vi "TEST Drop In.vi"(8 "error in (no error)":errorcluster, 10 "Queue Name":string="Main") -> (0 "error out":errorcluster)   [LabVIEW 2011]
doc: "This is the TEST VI that the user will leverage to test the drop in. \n\nAAL 9/09"
uses:
  Shared/QDMH Poly VIs/QDMH POLY Enqueue String.vi
panel:
  in  "Test 3":bool
  in  "Test 2":bool
  in  "Test 1":bool
  out "Message Display":string
  in  "Exit":bool
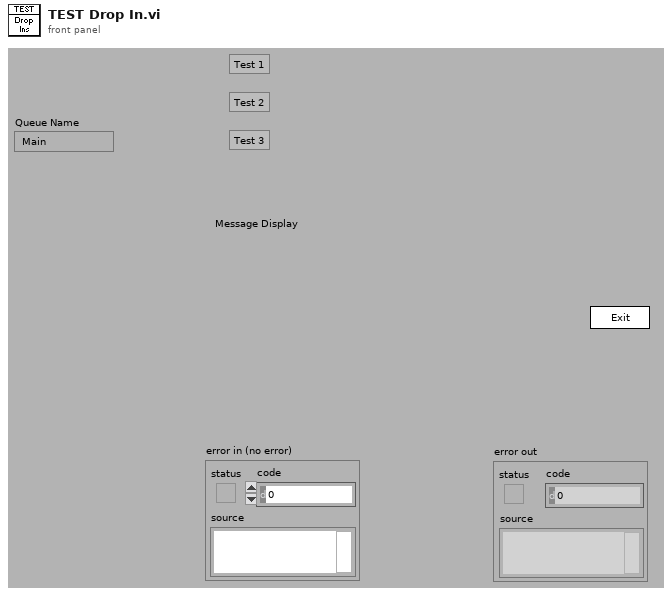
[diagram p1: front panel]
types:
  T1 = cluster{"Operator Name":string, "Current VI's Path":path, "Current VI's  Directory":path, "Queue Names":string[], "# VIs Launched":i32}
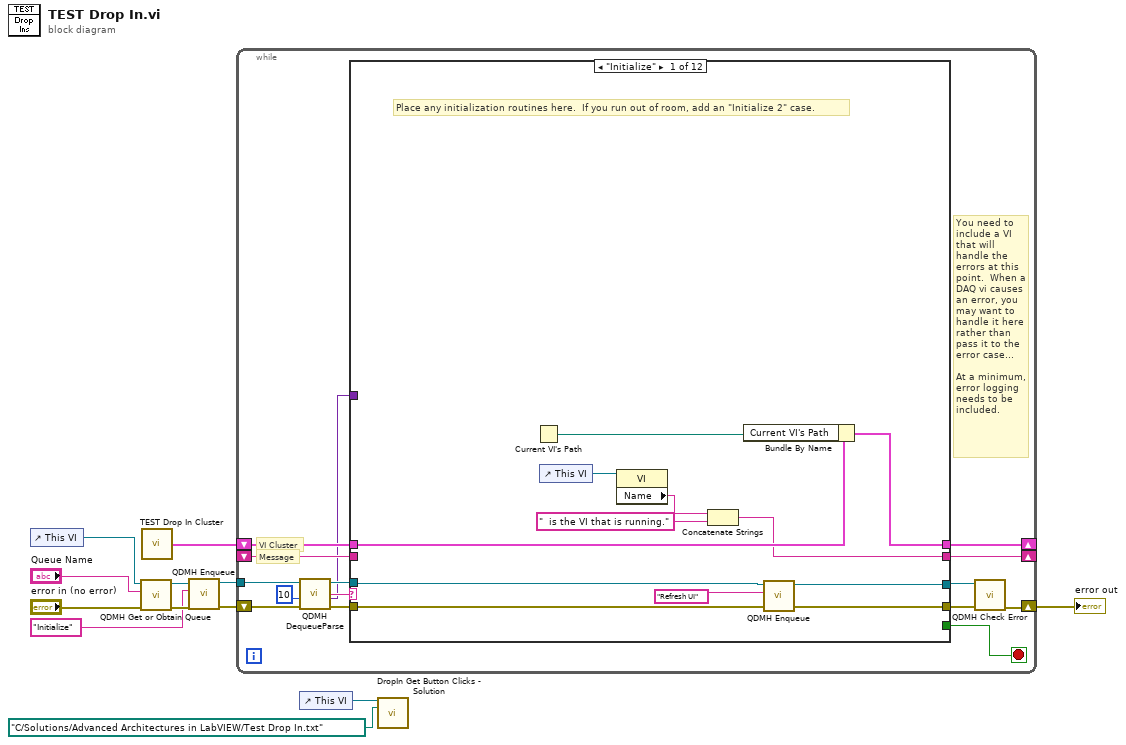
[diagram p0: block diagram]
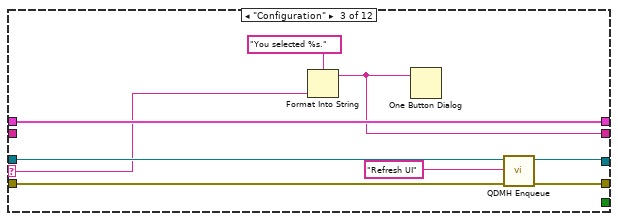
[diagram p3: hidden frame]
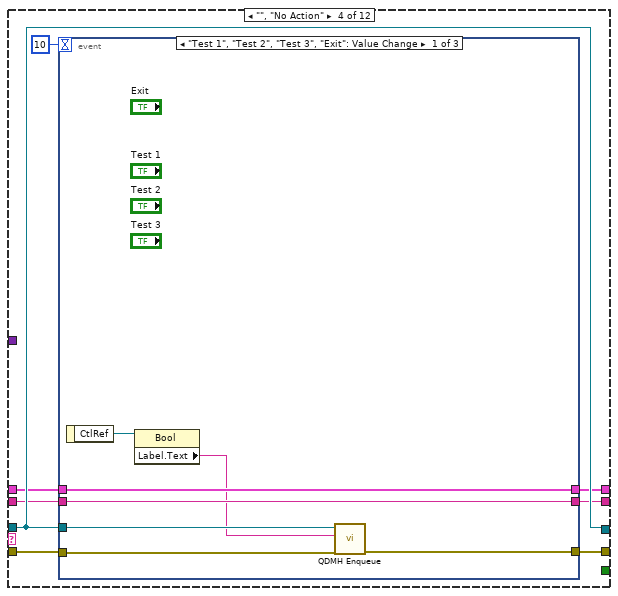
[diagram p4: hidden frame]
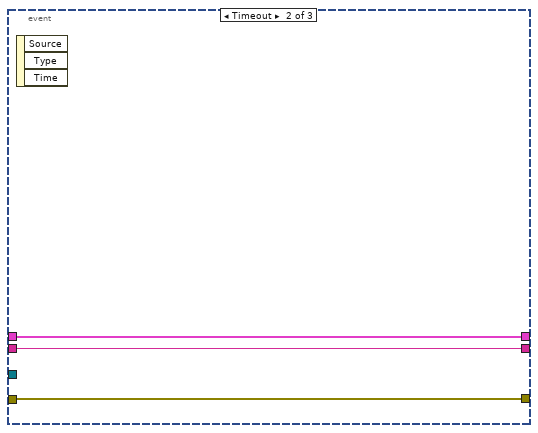
[diagram p5: hidden frame]
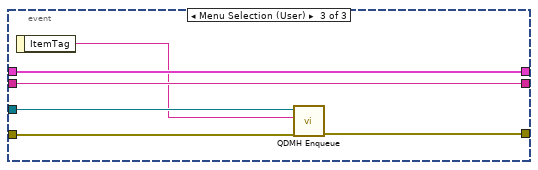
[diagram p6: hidden frame]
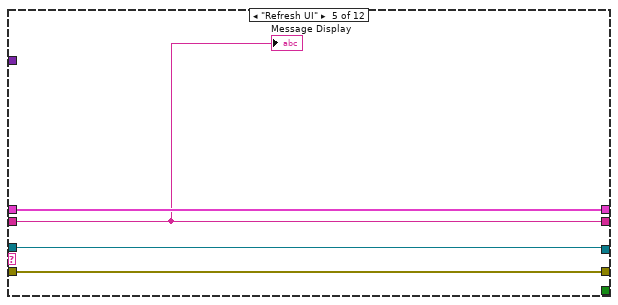
[diagram p7: hidden frame]
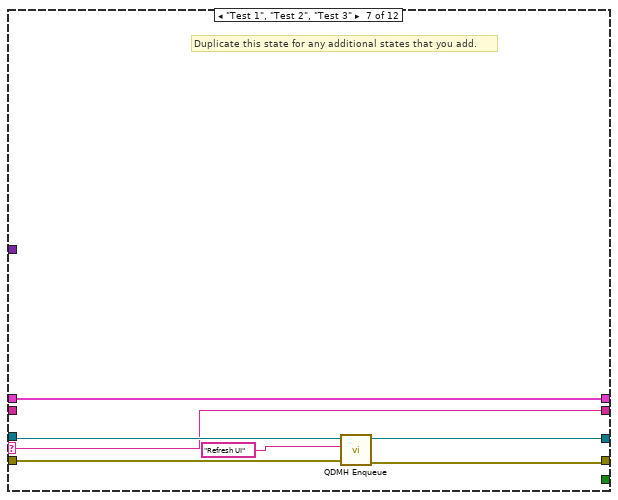
[diagram p9: hidden frame]
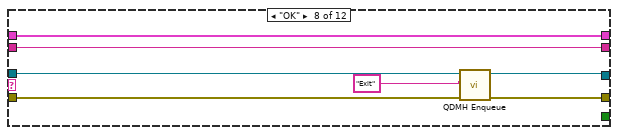
[diagram p10: hidden frame]
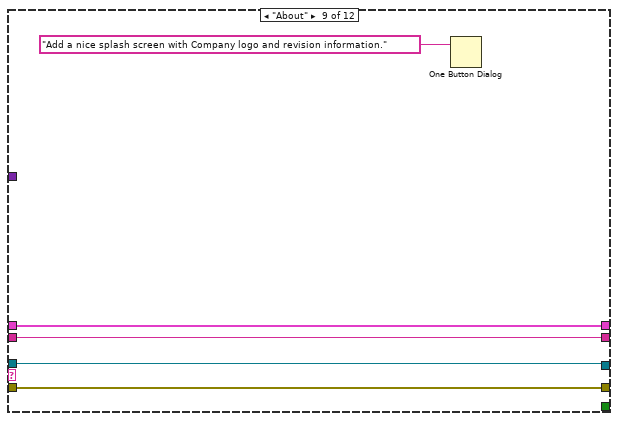
[diagram p11: hidden frame]
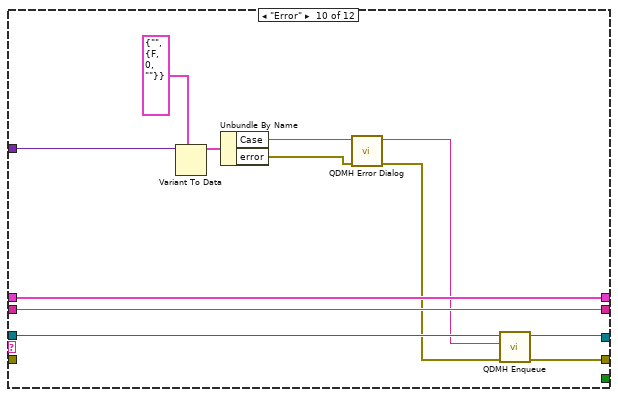
[diagram p12: hidden frame]
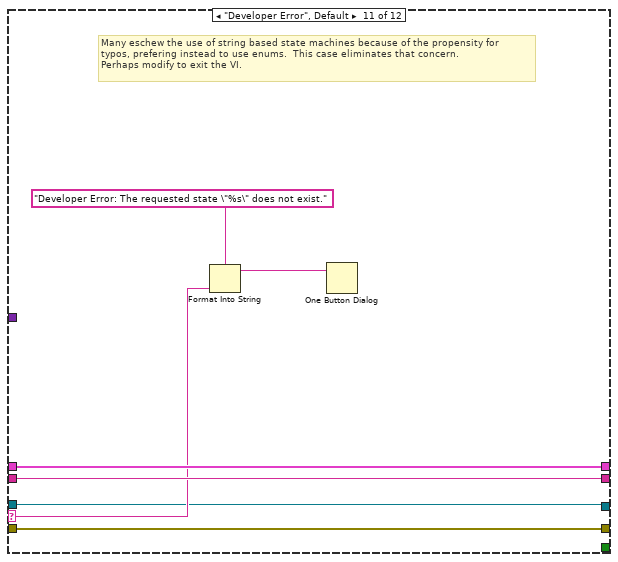
[diagram p13: hidden frame]
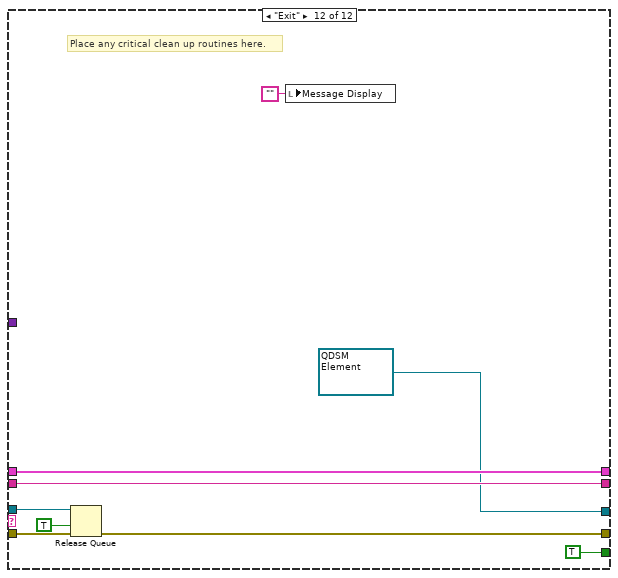
[diagram p14: hidden frame]
diagram:
  n1 = control-ref of="This VI"() -> (w4:refnum<vi>)
  n2 = call "QDMH Get or Obtain Queue.vi"("error in (no error)"="error in (no error)", "Queue Name"="Queue Name", "VI Refnum"=w4) -> ("error out"=w8:errorcluster, "queue out"=w11:refnum<queue>)  [unwired: 7 out]
  n3 = call "TEST Drop In Cluster.vi"() -> ("Cluster"=w10:T1)
  n4 = call-poly "QDMH Enqueue.vi"("error in (no error)"=w8, "State"="Initialize" ("element"), "queue"=w11) -> ("error out"=w9:errorcluster, "queue out"=w12:refnum<queue>)  [unwired: 7 out]
  n5 = while {
    tunnel: w12 -> [w22]
    shift-left: w10 -> [w23]
    shift-right: [w24] -> _
    shift-left: _ -> [w25]
    shift-right: [w26] -> _
    shift-right: [w16] -> w6
    shift-left: w9 -> [w17]
    stop <- w27 stop-if-true
    # "VI Cluster"
    # "Message"
    # "You need to include a VI that will handle the errors at this point.  When a DAQ vi causes an error, you may want to handle it here rather than pass it to the error case...\n\nAt a minimum,\nerror logging\nneeds to be \nincluded."
    n6 = call "QDMH DequeueParse.vi"("error in (no error)"=w17, "Timeout"=10 ("ms timeout (-1)"), "queue"=w22) -> ("error out"=w19:errorcluster, "Variant Data"=w13:variant, "State"=w18:string, "queue out"=w20:refnum<queue>)  [unwired: 5 out]
    n7 = case shown="\"Initialize\"" w18 {
      selector: w18 -> [_ _ w48 _ _ _ w87 _ _ _ w119 _]
      tunnel: w20 -> [w34 w40 w50 w60 w77 w81 w89 w98 w99 w113 w116 w128]
      tunnel: [_ _ _ _ _ _ _ _ _ _ _ TRUE] -> w27
      tunnel: [w32 w43 w49 w53 w79 w84 w87 w97 w103 w115 w122 w130] -> w26
      tunnel: w25 -> [_ w43 _ w54 w79 w84 _ w97 w103 w115 w122 w130]
      tunnel: [w38 w42 w52 w55 w80 w83 w91 w96 w102 w114 w121 w125] -> w24
      tunnel: w23 -> [w39 w42 w52 w56 w80 w83 w91 w96 w102 w114 w121 w125]
      tunnel: w19 -> [w36 w41 w47 w59 w78 w82 w90 w95 w100 _ w118 w127]
      tunnel: [w35 w41 w46 w58 w78 w82 w88 w94 w100 w112 w118 w124] -> w15
      tunnel: [w28 w40 w44 w60 w77 w81 w85 w93 w99 w111 w116 refnum<queue> refnum ("queue out")] -> w14
      tunnel: w13 -> [_ _ _ _ _ _ _ _ _ w106 _ _]
      frame "Initialize" {
        # "Place any initialization routines here.  If you run out of room, add an \"Initialize 2\" case."
        n8 = Current VI's Path() -> (path=w37:path)
        n9 = control-ref of="This VI"() -> (w31:refnum<vi>)
        n10 = property class="VI"(reference=w31) -> ("Name"=w30:string)  [unwired: 1 in, 2 out]
        n11 = Concatenate Strings(w30, "  is the VI that is running." ("string")) -> (w32:string)
        n12 = Bundle By Name(cluster=w39, "Current VI's Path"=w37) -> (w38:T1)
        n13 = call-poly "QDMH Enqueue.vi"("error in (no error)"=w36, "State"="Refresh UI" ("New State"), "queue"=w34) -> ("error out"=w35:errorcluster, "queue out"=w28:refnum<queue>)  [unwired: 7 out]
      }
      frame "Re-Initialize" {
        # "This case includes initialization functionality that may need to run again during the course of the VI"
      }
      frame "Configuration" {
        n14 = Format Into String(format string="You selected %s." ("Format String"), w48) -> (resulting string=w49:string)  [unwired: 2 in, 1 out]
        n15 = One Button Dialog(message=w49) -> ()  [unwired: 2 out]
        n16 = call-poly "QDMH Enqueue.vi"("error in (no error)"=w47, "State"="Refresh UI" ("New State"), "queue"=w50) -> ("error out"=w46:errorcluster, "queue out"=w44:refnum<queue>)  [unwired: 7 out]
      }
      frame "", "No Action" {
        n17 = event shown="[0] \"Test 1\", \"Test 2\", \"Test 3\", \"Exit\": Value Change" {
          selector: _ -> [_ _ _]
          dyn-events: _ -> [_ _ _]
          timeout: 10 -> [_ _ _]
          tunnel: w60 -> [w66 _ w76]
          tunnel: [w65 w70 w74] -> w58
          tunnel: w59 -> [w64 w70 w75]
          tunnel: w56 -> [w63 w69 w73]
          tunnel: [w63 w69 w73] -> w55
          tunnel: w54 -> [w62 w68 w72]
          tunnel: [w62 w68 w72] -> w53
          event "Test 1", "Test 2", "Test 3", "Exit": Value Change {
            n18 = event-data() -> ("CtlRef"=w67:refnum<vi>)  [unwired: 1 out]
            n19 = property class="Bool"(reference=w67) -> ("Label.Text"=w61:string)  [unwired: 1 in, 2 out]
            n20 = call-poly "QDMH Enqueue.vi"("error in (no error)"=w64, "State"=w61, "queue"=w66) -> ("error out"=w65:errorcluster)  [unwired: 8 out]
          }
          event Timeout {
            n21 = event-data() -> ()  [unwired: 4 out]
          }
          event Menu Selection (User) {
            n22 = event-data() -> ("ItemTag"=w71:string)  [unwired: 1 out]
            n23 = call-poly "QDMH Enqueue.vi"("error in (no error)"=w75, "State"=w71, "queue"=w76) -> ("error out"=w74:errorcluster)  [unwired: 8 out]
          }
        }
      }
      frame "Refresh UI" {
        "Message Display" <- w79
      }
      frame "<add states as needed>" {
        # "Duplicate this state for any additional states that you add."
      }
      frame "Test 1", "Test 2", "Test 3" {
        # "Duplicate this state for any additional states that you add."
        n24 = call-poly "QDMH Enqueue.vi"("error in (no error)"=w90, "State"="Refresh UI" ("element"), "queue"=w89) -> ("error out"=w88:errorcluster, "queue out"=w85:refnum<queue>)  [unwired: 7 out]
      }
      frame "OK" {
        n25 = call-poly "QDMH Enqueue.vi"("error in (no error)"=w95, "State"="Exit" ("New State"), "queue"=w98) -> ("error out"=w94:errorcluster, "queue out"=w93:refnum<queue>)  [unwired: 7 out]
      }
      frame "About" {
        n26 = One Button Dialog(message="Add a nice splash screen with Company logo and revision information.") -> ()  [unwired: 2 out]
      }
      frame "Error" {
        n27 = Variant To Data(type=cluster{"Case":string, "error":errorcluster} {"Case"="", "error"={"status"=FALSE, "code"=0, "source"=""}} ("QDSM Element"), Variant=w106) -> (data=w108:cluster{"Case":string, "error":errorcluster})  [unwired: 1 in, 1 out]
        n28 = Unbundle By Name(w108) -> ("Case"=w109:string, "error"=w110:errorcluster)
        n29 = call "QDMH Error Dialog.vi"("error"=w110, "Case Error Occured"=w109) -> ("error out (no error)"=w105:errorcluster, "Case to Execute"=w104:string)  [unwired: 8 out]
        n30 = call-poly "QDMH Enqueue.vi"("error in (no error)"=w105, "State"=w104, "queue"=w113) -> ("error out"=w112:errorcluster, "queue out"=w111:refnum<queue>)  [unwired: 7 out]
      }
      frame "Developer Error", Default {
        # "Many eschew the use of string based state machines because of the propensity for\ntypos, prefering instead to use enums.  This case eliminates that concern.\nPerhaps modify to exit the VI."
        n31 = Format Into String(format string="Developer Error: The requested state \"%s\" does not exist." ("message"), w119) -> (resulting string=w117:string)  [unwired: 2 in, 1 out]
        n32 = One Button Dialog(message=w117) -> ()  [unwired: 2 out]
      }
      frame "Exit" {
        # "Place any critical clean up routines here."
        n33 = Release Queue(queue=w128, force destroy? (F)=TRUE, error in (no error)=w127) -> (error out=w124:errorcluster)  [unwired: 2 out]
        n34 = local write "Message Display"("") -> ()
      }
    }
    n35 = call "QDMH Check Error.vi"("error in (no error)"=w15, "queue"=w14) -> ("error out"=w16:errorcluster)  [unwired: 2 in, 7 out]
  }
  "error out" <- w6
  n36 = control-ref of="This VI"() -> (w2:refnum<vi>)
  n37 = call "DropIn Get Button Clicks - Solution.vi"("VI Refnum"=w2, "file path"=path "C:/Solutions/Advanced Architectures in LabVIEW/Test Drop In.txt") -> ()  [unwired: 13 in, 1 out]
